vi "Receive Value Change Event.vi"(8 "error in (no error)":errorcluster, 10 "ValueChangeMsg":refnum<class "ValueChangeMsg.lvclass">, 11 "User Manager View In":refnum<class "User Manager View.lvclass">) -> (0 "error out":errorcluster, 3 "User Manager View Out":refnum<class "User Manager View.lvclass">)   [LabVIEW 2017, in "User Manager View.lvlib" / "User Manager View.lvclass"]
doc: "<License>\nCopyright © 2017 Composed Systems, LLC | All rights reserved\nwww.composed.io\n\nAuthor: Ethan Stern <ethan.stern@composed.io>\n\nThis software is provided \"AS IS\" WITHOUT WARRANTIES, either express or implied, AND IS FOR EDUCATIONAL PURPOSES ONLY.\n</License>"
uses:
  <vilib>/gpm_packages/@cs/User Manager App/User Manager View/User Manager View/User Manager View.lvclass
  C:/Program Files/National Instruments/LabVIEW 2017/vi.lib/ActorFramework/Actor/Actor.lvclass
  <vilib>/gpm_packages/@cs/mva-viewable/Source/ActorEvents/IEventAggregator Messages/ValueChangeMsg/ValueChangeMsg.lvclass
  <vilib>/ActorFramework/Actor/Actor.lvclass/Actor.ctl
  <vilib>/ActorFramework/Message Enqueuer/Message Enqueuer.lvclass/Message Enqueuer.ctl
  <vilib>/gpm_packages/@cs/mva-viewable/Source/ActorEvents/IEventAggregator Messages/ValueChangeMsg/ValueChangeMsg.lvclass/ValueChangeMsg.ctl
  <vilib>/gpm_packages/@cs/User Manager App/User Manager View/User Manager View Messages/Edit User Msg/Edit User Msg.lvclass/Edit User Msg.ctl
  <vilib>/gpm_packages/@cs/User Manager App/User Manager View/User Manager View Messages/Pick User Msg/Pick User Msg.lvclass/Pick User Msg.ctl
  <vilib>/ActorFramework/Message Enqueuer/Init from Existing Queue.vi
  <vilib>/ActorFramework/Message Enqueuer/Enqueue.vi
  <vilib>/gpm_packages/@cs/User Manager App/User Manager View/User Manager View Messages/Remove User Msg/Remove User Msg.lvclass
  C:/Program Files/National Instruments/LabVIEW 2017/vi.lib/ActorFramework/Message/Message.lvclass
  <vilib>/gpm_packages/@cs/User Manager App/User Manager View/User Manager View Messages/Add User Msg/Add User Msg.lvclass
  <vilib>/gpm_packages/@cs/User Manager App/User Manager View/User Manager View Messages/Edit User Msg/Edit User Msg.lvclass
  <vilib>/gpm_packages/@cs/User Manager App/User Manager View/User Manager View Messages/Undo Msg/Undo Msg.lvclass
  <vilib>/gpm_packages/@cs/User Manager App/User Manager View/User Manager View Messages/Save Msg/Save Msg.lvclass
  <vilib>/gpm_packages/@cs/User Manager App/User Manager View/User Manager View Messages/Pick User Msg/Pick User Msg.lvclass
  <vilib>/ActorFramework/Message Priority Queue/Priority Enqueue.vi
  <vilib>/ActorFramework/Message Enqueuer/Message Enqueuer.lvclass
  <vilib>/gpm_packages/@cs/mva-viewable/Source/IViewable/IViewable/IViewable.lvclass
  <vilib>/ActorFramework/Actor/Actor.lvclass
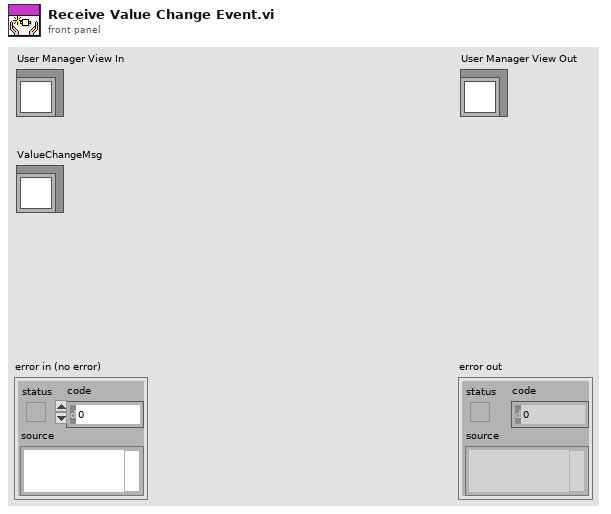
[diagram p1: front panel]
types:
  T1 = cluster{"User name":string, "Password":string, "User Level":string}
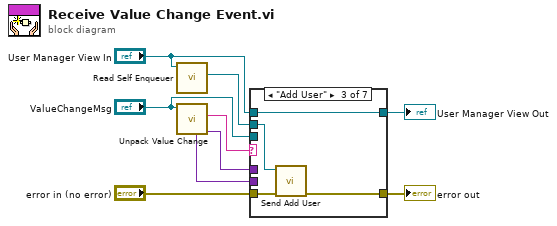
[diagram p0: block diagram]
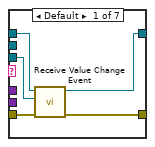
[diagram p2: hidden frame]
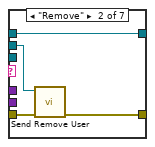
[diagram p3: hidden frame]
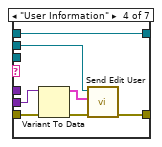
[diagram p4: hidden frame]
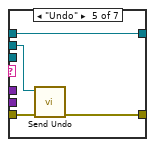
[diagram p5: hidden frame]
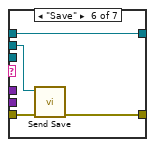
[diagram p6: hidden frame]
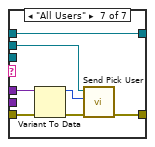
[diagram p7: hidden frame]
diagram:
  n1 = call <vilib>:"Read Self Enqueuer.vi"("Actor"="User Manager View In") -> ("Self Enqueuer"=w1:refnum<class "Message Enqueuer.lvclass">)  [unwired: 10 in]
  n2 = call <vilib>:"Unpack Value Change.vi"("ValueChangeMsg"="ValueChangeMsg") -> ("New Value"=w4:variant, "Control Label"=w5:string, "Old Value"=w3:variant)  [unwired: 6 in, 2 out]
  n3 = case shown="\"Add User\"" w5 {
    tunnel: [w14 w15 w19 w23 w30 w34 w38] -> w9
    tunnel: [w13 w18 w22 w29 w33 w37 w44] -> w8
    tunnel: "error in (no error)" -> [w12 w16 w20 w25 w31 w35 w40]
    tunnel: "ValueChangeMsg" -> [w11 _ _ _ _ _ _]
    tunnel: "User Manager View In" -> [w10 w18 w22 w29 w33 w37 w44]
    tunnel: w4 -> [_ _ _ _ _ _ w43]
    tunnel: w3 -> [_ _ _ w27 _ _ _]
    tunnel: w1 -> [_ w17 w21 w28 w32 w36 w41]
    frame Default {
      n4 = call-parent "Receive Value Change Event.vi"("error in (no error)"=w12, "ValueChangeMsg"=w11, "IViewable In"=w10) -> ("error out"=w14:errorcluster, "IViewable Out"=w13:refnum<class "User Manager View.lvclass">)  [unwired: 7 in]
    }
    frame "Remove" {
      n5 = call <vilib>:"Send Remove User.vi"("error in (no error)"=w16, "Message Enqueuer"=w17) -> ("error out"=w15:errorcluster)  [unwired: 8 in, 1 out]
    }
    frame "Add User" {
      n6 = call <vilib>:"Send Add User.vi"("error in (no error)"=w20, "Message Enqueuer"=w21) -> ("error out"=w19:errorcluster)  [unwired: 8 in, 1 out]
    }
    frame "User Information" {
      n7 = Variant To Data(error in=w25, Variant=w27) -> (data=w26:T1, error out=w24:errorcluster)  [unwired: 1 in]
      n8 = call <vilib>:"Send Edit User.vi"("error in (no error)"=w24, "OldVal"=w26, "Message Enqueuer"=w28) -> ("error out"=w23:errorcluster)  [unwired: 7 in, 1 out]
    }
    frame "Undo" {
      n9 = call <vilib>:"Send Undo.vi"("error in (no error)"=w31, "Message Enqueuer"=w32) -> ("error out"=w30:errorcluster)  [unwired: 8 in, 1 out]
    }
    frame "Save" {
      n10 = call <vilib>:"Send Save.vi"("error in (no error)"=w35, "Message Enqueuer"=w36) -> ("error out"=w34:errorcluster)  [unwired: 8 in, 1 out]
    }
    frame "All Users" {
      n11 = Variant To Data(error in=w40, Variant=w43) -> (data=w42:i32, error out=w39:errorcluster)  [unwired: 1 in]
      n12 = call <vilib>:"Send Pick User.vi"("error in (no error)"=w39, "NewVal"=w42, "Message Enqueuer"=w41) -> ("error out"=w38:errorcluster)  [unwired: 7 in, 1 out]
    }
  }
  "error out" <- w9
  "User Manager View Out" <- w8
